vi "Configure Computation Constant.vi"(0 "VISA resource name":refnum<visa-resource-name>, 5 "Constant Number (001)":string="001", 7 "Constant Value (0.0000E+0)":dbl min=-9.9999e+29 max=9.9999e+29 step=0.0001 format="%#_8g", 11 "error in (no error)":errorcluster) -> (4 "VISA resource name out":refnum<visa-resource-name>, 6 "Constant Number":string, 15 "error out":errorcluster)   [LabVIEW 2020, in "Yokogawa GX Series.lvlib"]
doc: "Sets the computation constant.\n\nCommand: SKConst"
uses:
  <instrlib>/Yokogawa GX Series/Yokogawa GX Series.lvlib
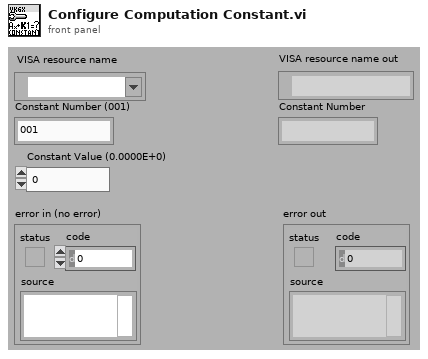
[diagram p1: front panel]
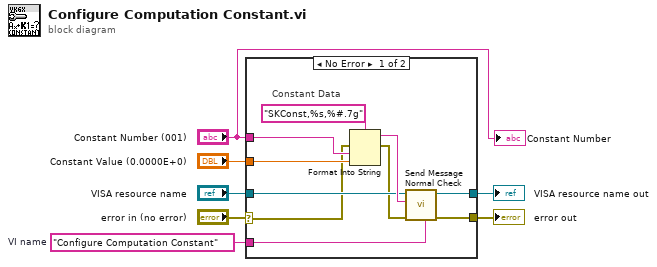
[diagram p0: block diagram]
diagram:
  w6 = "Configure Computation Constant"  # VI name
  n1 = case shown="No Error" "error in (no error)" {
    selector: "error in (no error)" -> [w8 w18]
    tunnel: "VISA resource name" -> [w15 w19]
    tunnel: w6 -> [w13 _]
    tunnel: "Constant Value (0.0000E+0)" -> [w12 _]
    tunnel: [w11 w19] -> w4
    tunnel: [w10 w18] -> w3
    tunnel: "Constant Number (001)" -> [w9 _]
    frame No Error {
      # "Constant Data"
      n2 = Format Into String(format string="SKConst,%s,%#.7g", error in=w8, w9, w12) -> (resulting string=w16:string, error out=w14:errorcluster)  [unwired: 1 in]
      n3 = call <instrlib>:"Send Message Normal Check.vi"("Source (\"\")"=w13, "error in (no error)"=w14, "Send Message (\"\")"=w16, "VISA resource name"=w15) -> ("error out"=w10:errorcluster, "VISA resource name out"=w11:refnum<visa-resource-name>)  [unwired: 2 in, 4 out]
    }
    frame Error {
    }
  }
  "error out" <- w3
  "VISA resource name out" <- w4
  "Constant Number" <- "Constant Number (001)"
